vi "LVClass_WavefrontCorrector Move to Absolute Position.vi"(0 "WavefrontCorrector in":refnum<class "WavefrontCorrector.lvclass">, 5 "Absolute Positions":T1, 11 "error in (no error)":errorcluster) -> (4 "WavefrontCorrector out":refnum<class "WavefrontCorrector.lvclass">, 15 "error out":errorcluster)   [LabVIEW 2020, in "WavefrontCorrector.lvclass"]
doc: "Move to requested absolute positions, clip according to current preferences.\n\n--------------------------------------------------------------------------------\n\n<B>correctorIn </B> : WavefrontCorrector object.\n<B>correctorOut </B> : WavefrontCorrector object.\n<B>position </B> : Requested absolutes positions.\n<B>ErrorIn </B> : Error\n<B>ErrorOut </B> : Error\n\n--------------------------------------------------------------------------------"
uses:
  WavefrontCorrector.lvclass
  Controls/Wavefront Corrector Position.ctl
  WavefrontCorrector.lvclass/WavefrontCorrector.ctl
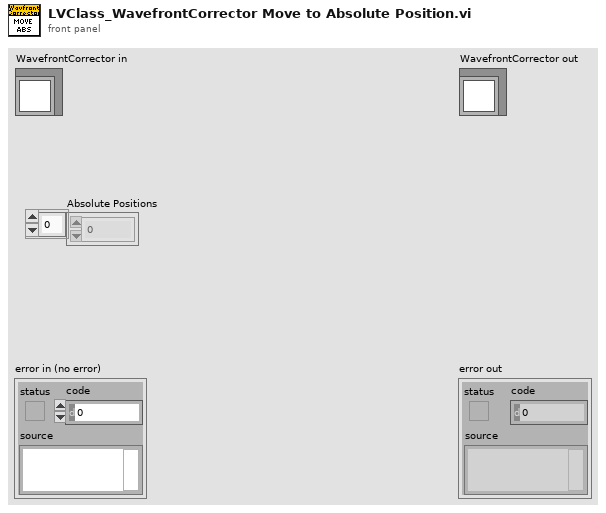
[diagram p1: front panel]
types:
  T1 = typedef "Wavefront Corrector Position.ctl" = sgl[]
  T2 = typedef "ClassID.ctl" = i64
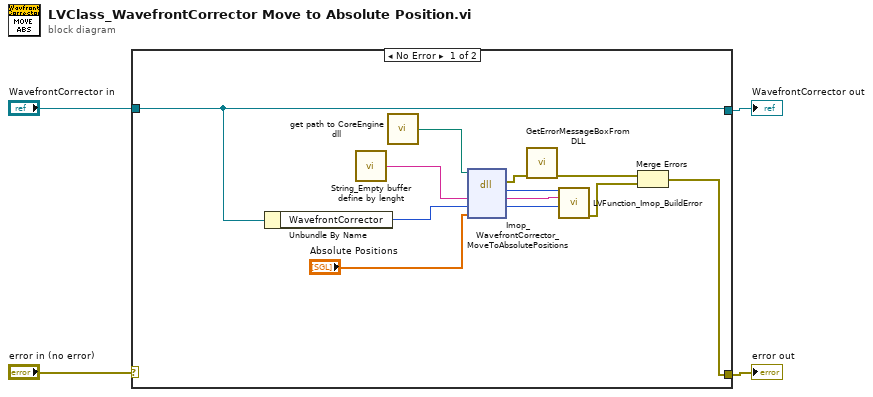
[diagram p0: block diagram]
diagram:
  n1 = case shown="No Error" "error in (no error)" {
    selector: "error in (no error)" -> [_ w18]
    tunnel: [w8 w18] -> w1
    tunnel: [w7 w17] -> w2
    tunnel: "WavefrontCorrector in" -> [w7 w17]
    frame No Error {
      n2 = Unbundle By Name(w7) -> ("WavefrontCorrector"=w9:T2)
      n3 = call "String_Empty buffer define by lenght.vi"() -> ("Empty buffer"=w14:string)  [unwired: 1 in]
      n4 = call "get path to CoreEngine dll.vi"() -> ("path to wavekit library"=w13:path)  [unwired: 14 in, 1 out]
      n5 = dll-call lib="D:/soft/HASO_v3/SVN_trunk/ImOpCoreEngine4_LV2011/DLLs/c_interface_vc100.dll" fn="Imop_WavefrontCorrector_MoveToAbsolutePositions"(path in=w13, "message"=w14, "WavefrontCorrection"=w9, "Absolute Position"="Absolute Positions") -> (error out=w12:errorcluster, "return type"=w16:i32, "message"=w15:string, "WavefrontCorrection"=w5:i64)  [unwired: 3 in, 1 out]
      n6 = call "GetErrorMessageBoxFromDLL.vi"("error IN"=w12) -> ("error OUT"=w11:errorcluster)  [unwired: 10 in]
      n7 = call "LVFunction_Imop_BuildError.vi"("code"=w16, "String to Prepend to source (\"\")"=w15, "Adresse"=w5) -> ("error out"=w10:errorcluster)  [unwired: 12 in]
      n8 = Merge Errors(w11, w10) -> (w8:errorcluster)
    }
    frame Error {
    }
  }
  "error out" <- w1
  "WavefrontCorrector out" <- w2
